vi "TAT_Varient Creater_Station2.vi"(8 "error in (no error)":errorcluster) -> (0 "error out":errorcluster)   [LabVIEW 2017]
uses:
  <vilib>/Utility/miscctls.llb/LVRangeTypeDef.ctl
  <vilib>/addons/database/Connection.llb/Conn ObjectReference.ctl
  <vilib>/Utility/miscctls.llb/LVRowAndColumnUnsignedTypeDef.ctl
  cc04d7d6-45d9-4bf1-9dd6-3a820b5b8d83.vi
  <vilib>/Utility/config.llb/Read Key (I32).vi
  <vilib>/Utility/config.llb/Read Key (String).vi
  <vilib>/Utility/config.llb/Read Key (Boolean).vi
  <vilib>/Utility/config.llb/Write Key (U32).vi
  <vilib>/Utility/config.llb/Write Key (String).vi
  <vilib>/Utility/config.llb/Write Key (Boolean).vi
  <vilib>/Utility/config.llb/NI_LVConfig.lvlib
  <vilib>/addons/database/NI_Database_API.lvlib
panel:
  in  "STATION 1\nBYPASS":bool
  in  "Vertical Slider Control":dbl(slide)=1.0 scale=0.0..-2.0
  in  "CANCLE 3":bool
  in  "PRINTING":bool
  in  "Manual print":bool
  in  "Cancle 2":bool
  in  "Delete Button":bool
  in  "Cancle":bool
  in  "Save Button":bool
  in  "TORISHI CODE":string
  in  "PART NUMBER":string
  in  "Delete Square":bool
  in  "EDIT & SAVE":bool
  out "Varient Details":string[][](table)
  in  "BATCH SIZE":u16=1 min=1 max=100 step=1
  in  "VARIENT NUMBER":u16=1 min=1 max=100 step=1
  in  "HOME":bool
  in  "UPDATE TABLE":bool
  in  "PART NAME":string(combo)
  # "Varient Creater Station 2"
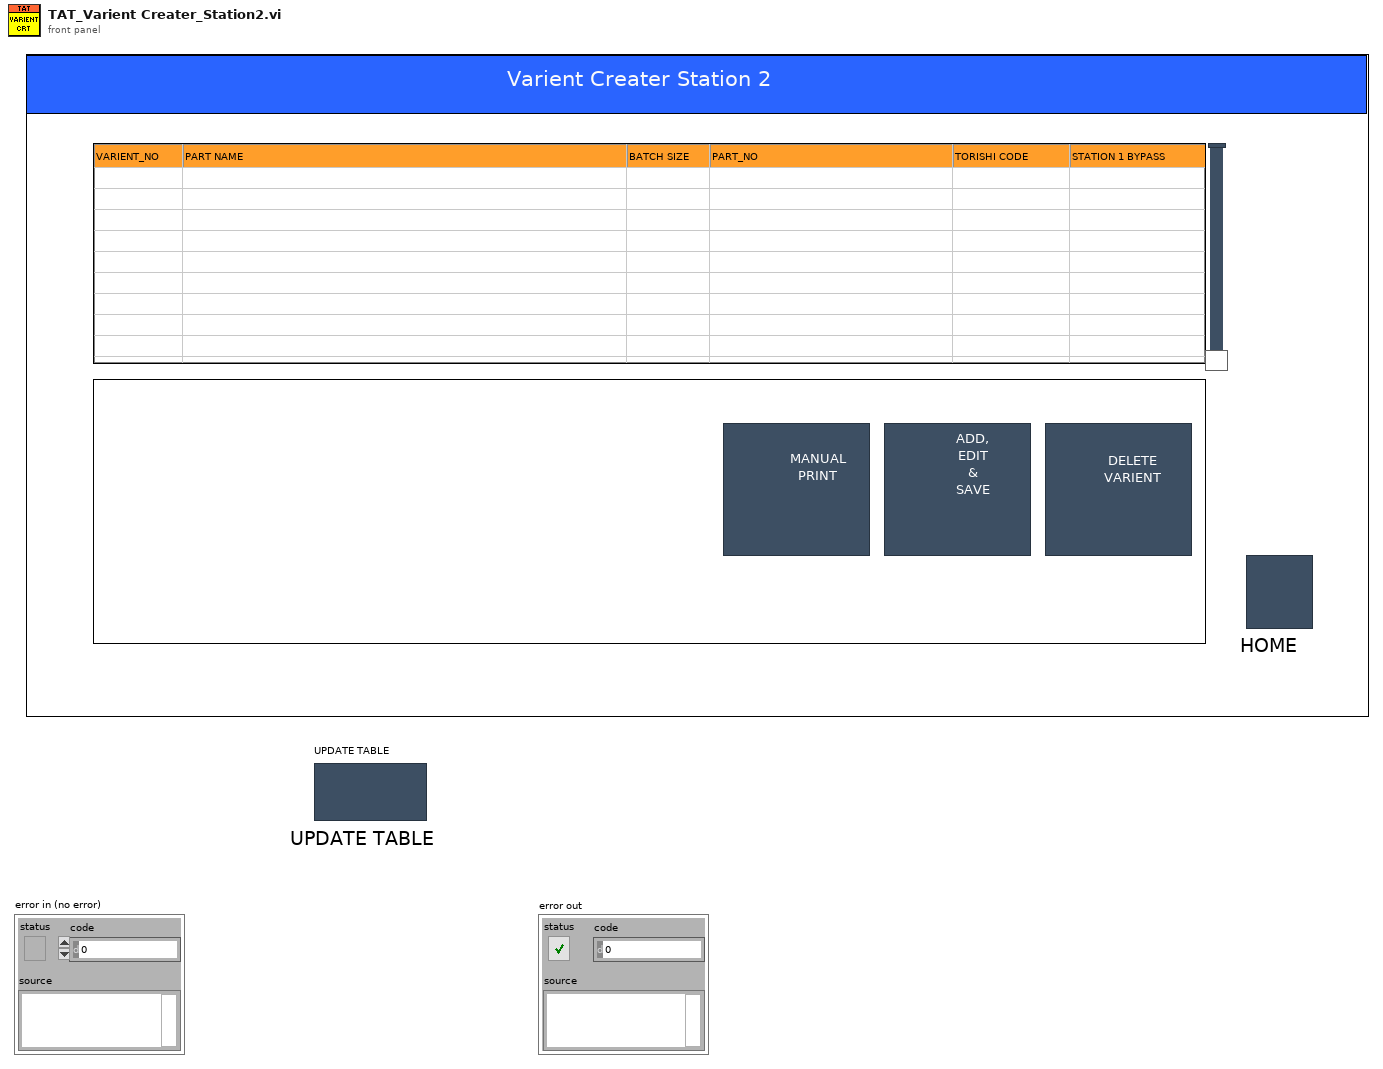
[diagram p1: front panel]
types:
  T1 = enum8{"Enabled", "Disabled", "Disabled and Grayed Out"}
  T2 = enum32{"invalid app kind", "Development System", "Run Time System", "Student Edition", "Embedded LabVIEW", "Evaluation", "Custom"}
  T3 = typedef "NI_LVConfig.lvlib/Config Data RefNum.ctl" = refnum<k1>
  T4 = typedef "LVRangeTypeDef.ctl" = cluster{"Minimum":dbl, "Maximum":dbl, "Increment":dbl, "Minor Increment":dbl, "Start":dbl}
  T5 = typedef "NI_Database_API.lvlib/Conn ObjectReference.ctl" = refnum<k1>
  T6 = cluster{"Varient number":u16, "Part name":string, "connection reference":T5, "Batch_Size":u16, "PART_NO":string, "TORISHI_CODE":string, "scanner com":refnum<visa-resource-name>, "Part Name List":string[], "Varient path":path, "Current Varient path":path, "Communication path":path, "Package path":path, "Part PRN path":path, "Station2 printer IP":string, "Station1 printer IP":string, "Current Serial Number":string, "Station1_QR":string, "Serial_Number":path, "PRIVIOUS code":string[], "Barcode station2 log":string, "Barcode station2 Up":string, "HARNESS CODE":string, "Station 1 Bypass":bool}
  T7 = enum16{"open", "replace", "create", "open or create", "replace or create", "replace or create with confirmation"}
  T8 = typedef "LVRowAndColumnUnsignedTypeDef.ctl" = cluster{"Row":u32, "Column":u32}
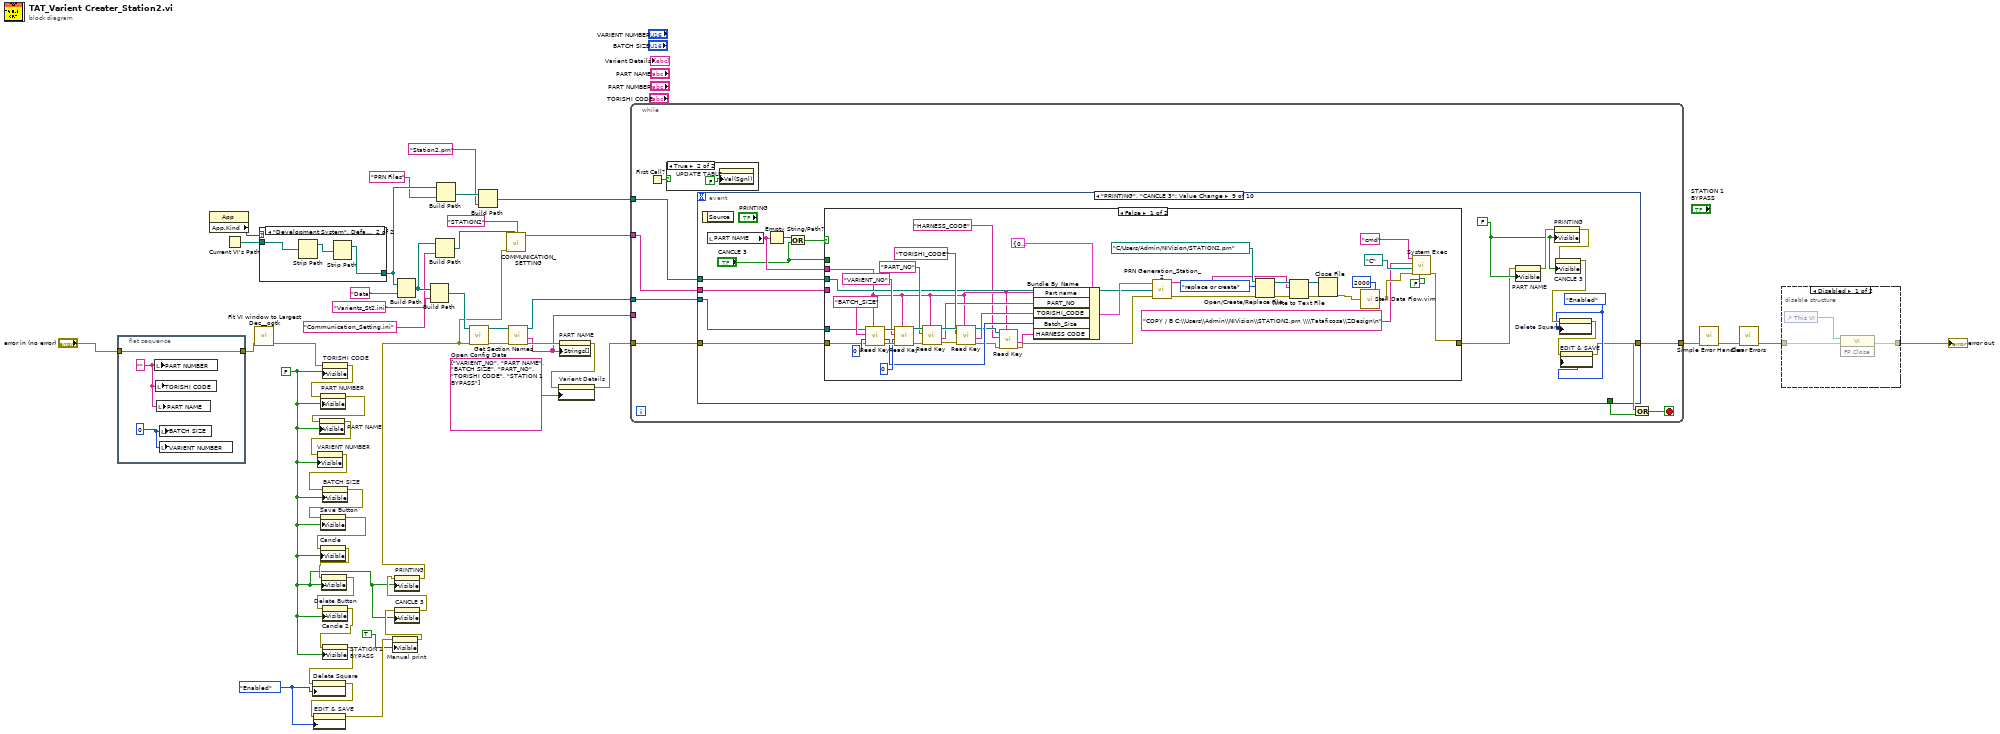
[diagram p0: block diagram]
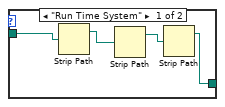
[diagram p3: hidden frame]
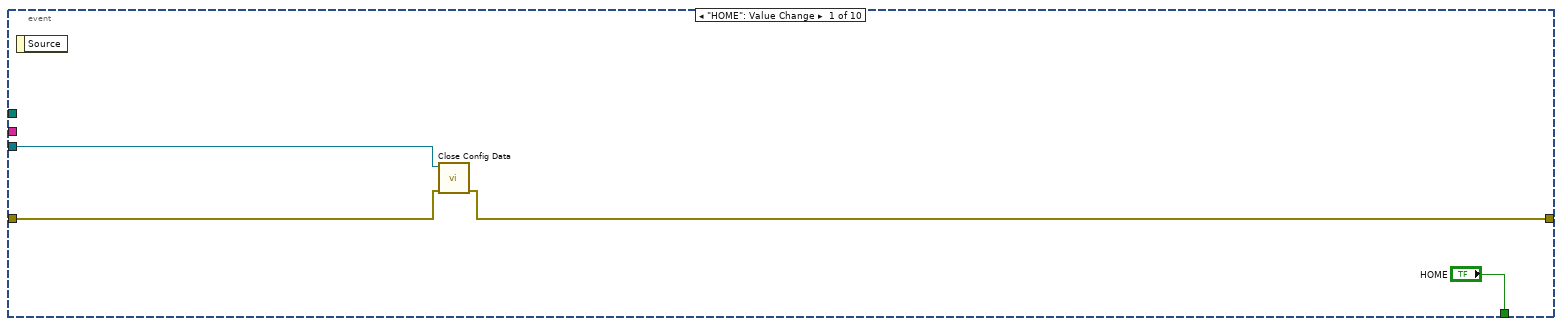
[diagram p5: hidden frame]
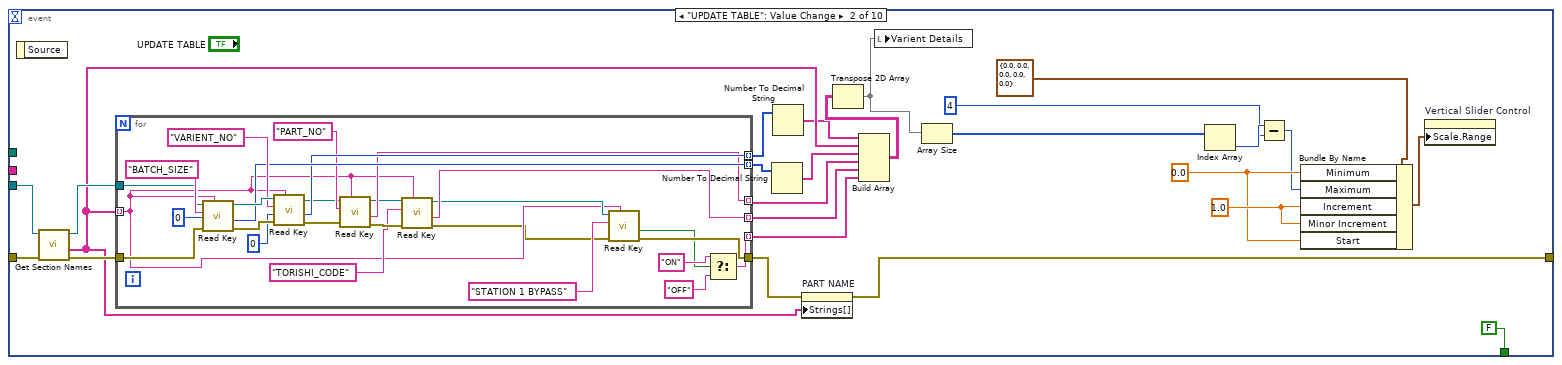
[diagram p6: hidden frame]
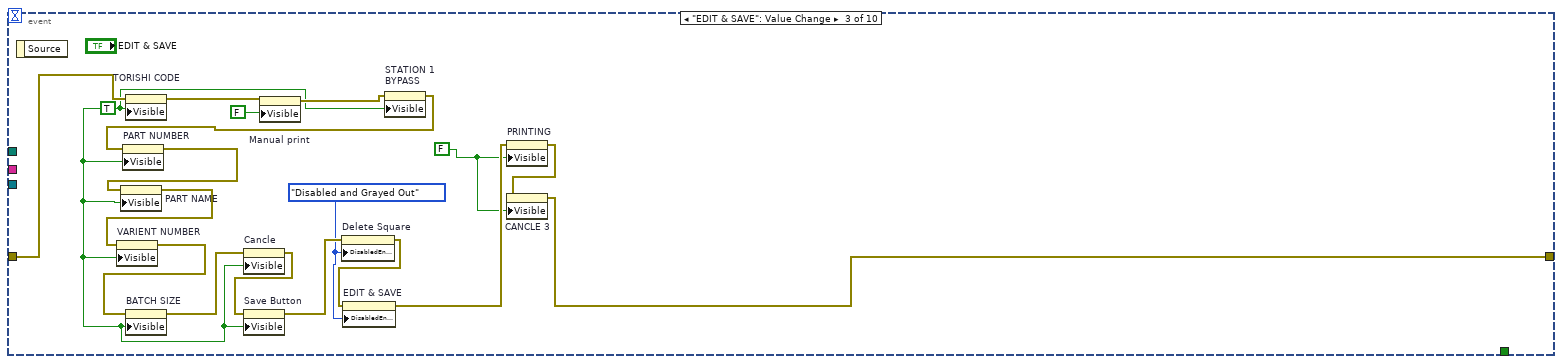
[diagram p7: hidden frame]
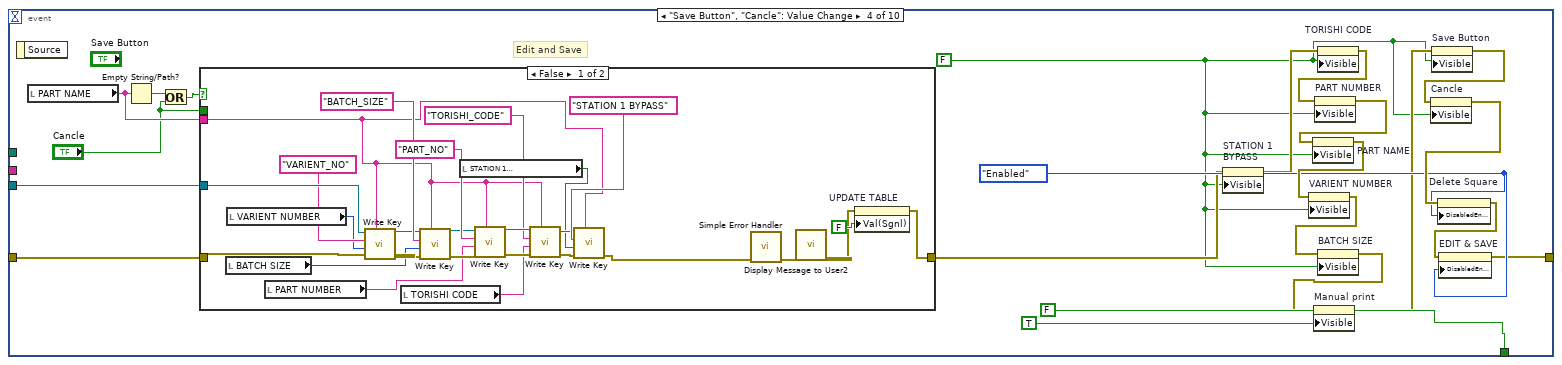
[diagram p8: hidden frame]
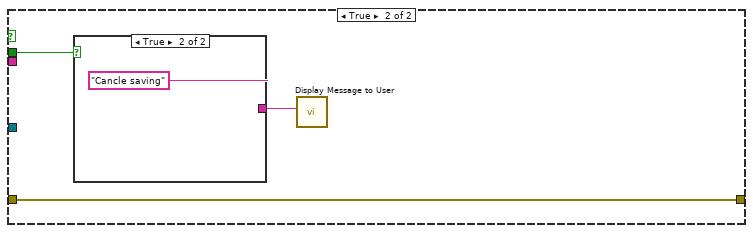
[diagram p9: hidden frame]
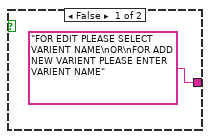
[diagram p10: hidden frame]
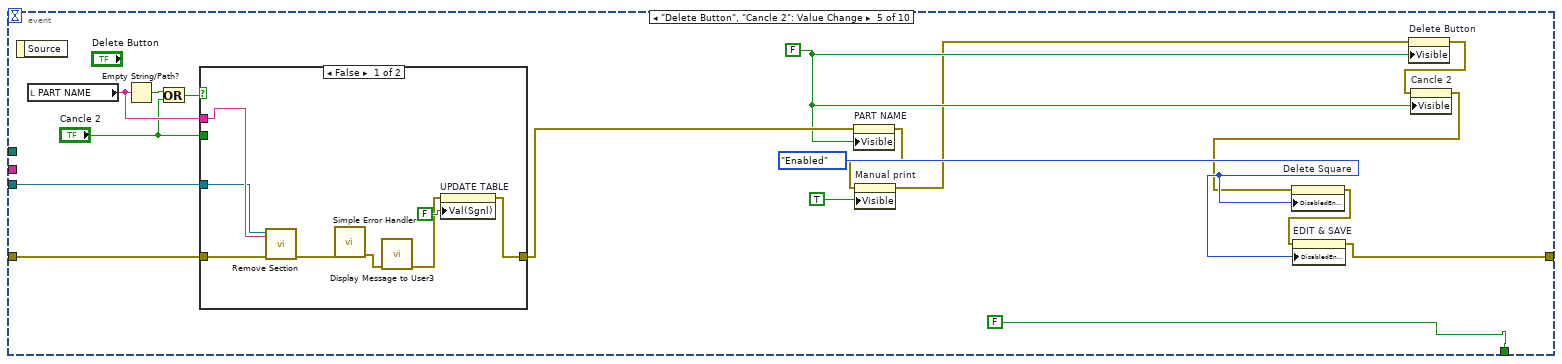
[diagram p11: hidden frame]
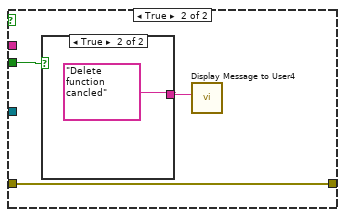
[diagram p12: hidden frame]
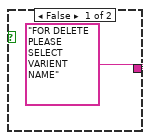
[diagram p13: hidden frame]
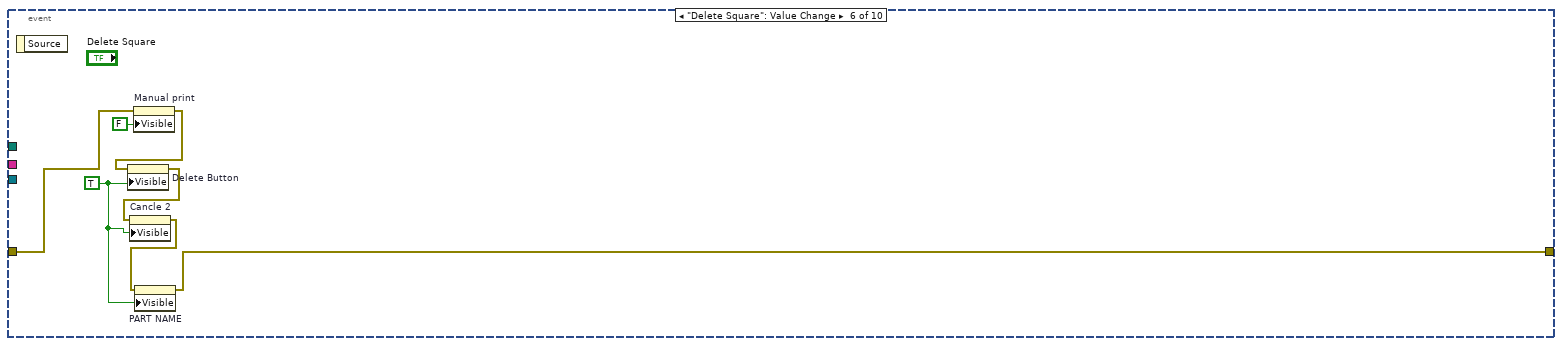
[diagram p14: hidden frame]
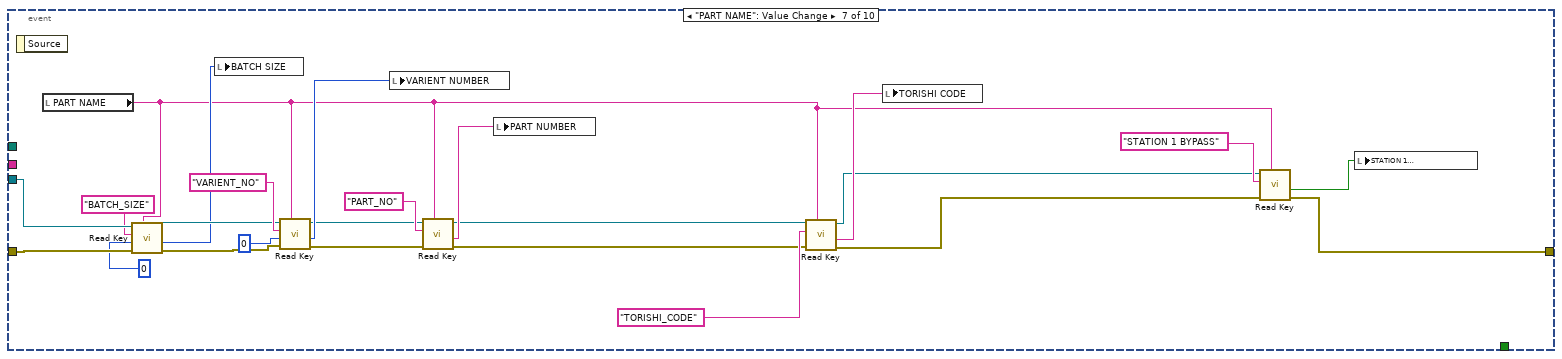
[diagram p15: hidden frame]
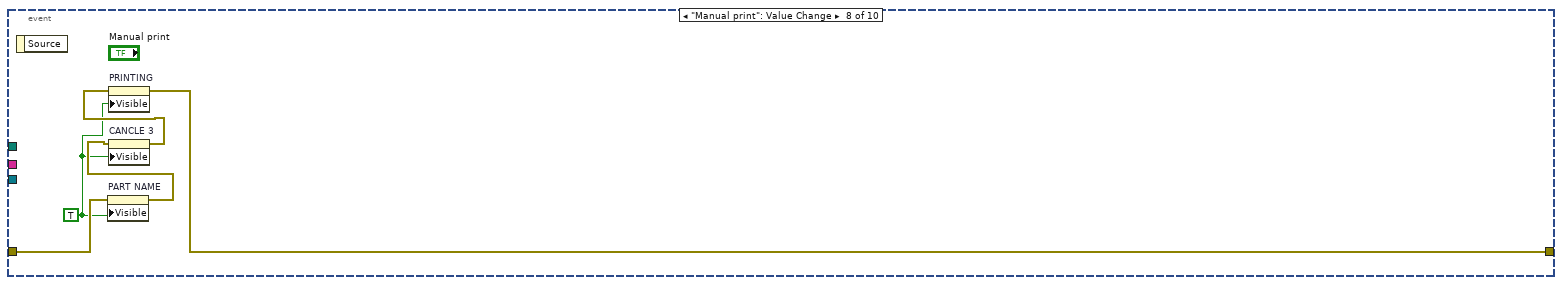
[diagram p16: hidden frame]
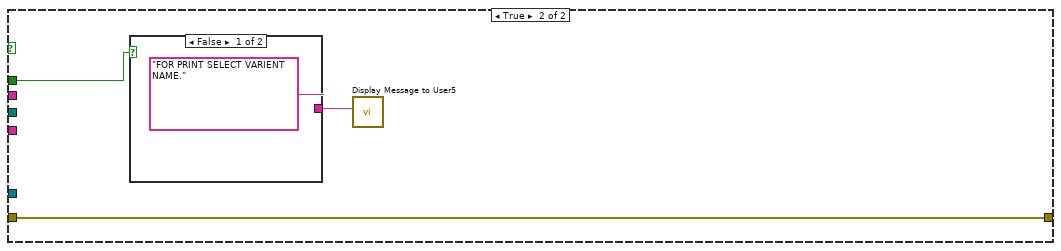
[diagram p17: hidden frame]
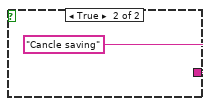
[diagram p18: hidden frame]
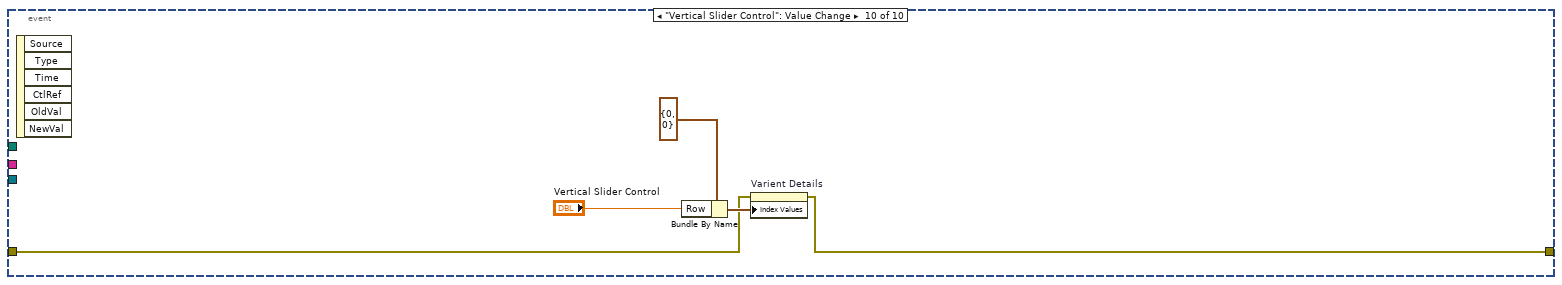
[diagram p19: hidden frame]
diagram:
  w22 = T1."Enabled" ("Disabled")
  w3 = FALSE
  n1 = flat-sequence {
    tunnel: [w49] -> w30
    tunnel: "error in (no error)" -> [w49]
    frame #0 {
      w50 = u16 0 ("BATCH SIZE")
      w51 = "" ("PART NUMBER")
      n2 = local write "PART NUMBER"(w51) -> ()
      n3 = local write "TORISHI CODE"(w51) -> ()
      n4 = local write "PART NAME"(w51) -> ()
      n5 = local write "BATCH SIZE"(w50) -> ()
      n6 = local write "VARIENT NUMBER"(w50) -> ()
    }
  }
  n7 = property class="App"() -> ("App.Kind"=w43:T2)  [unwired: 2 in, 2 out]
  n8 = Current VI's Path() -> (path=w44:path)
  n9 = call <userlib>:"Fit VI window to Largest Dec__ogtk.vi"("error in (no error)"=w30) -> ("error out"=w25:errorcluster)  [unwired: 5 in, 1 out]
  n10 = case shown="\"Development System\", Default" w43 {
    tunnel: w44 -> [w53 w57]
    tunnel: [w52 w56] -> w8
    frame "Run Time System" {
      n11 = Strip Path(path=w53) -> (stripped path=w55:path)  [unwired: 1 out]
      n12 = Strip Path(path=w55) -> (stripped path=w54:path)  [unwired: 1 out]
      n13 = Strip Path(path=w54) -> (stripped path=w52:path)  [unwired: 1 out]
    }
    frame "Development System", Default {
      n14 = Strip Path(path=w57) -> (stripped path=w58:path)  [unwired: 1 out]
      n15 = Strip Path(path=w58) -> (stripped path=w56:path)  [unwired: 1 out]
    }
  }
  n16 = property on="TORISHI CODE" class="Str"(error in=w25, "Visible"=w3) -> (error out=w29:errorcluster)  [unwired: 1 in, 1 out]
  n17 = property on="PART NUMBER" class="Str"(error in=w29, "Visible"=w3) -> (error out=w28:errorcluster)  [unwired: 1 in, 1 out]
  n18 = property on="PART NAME" class="CmbBox"(error in=w28, "Visible"=w3) -> (error out=w27:errorcluster)  [unwired: 1 in, 1 out]
  n19 = property on="VARIENT NUMBER" class="DigNum (strict)"(error in=w27, "Visible"=w3) -> (error out=w26:errorcluster)  [unwired: 1 in, 1 out]
  n20 = property on="BATCH SIZE" class="DigNum (strict)"(error in=w26, "Visible"=w3) -> (error out=w24:errorcluster)  [unwired: 1 in, 1 out]
  n21 = property on="Save Button" class="Bool"(error in=w24, "Visible"=w3) -> (error out=w21:errorcluster)  [unwired: 1 in, 1 out]
  n22 = property on="Cancle" class="Bool"(error in=w21, "Visible"=w3) -> (error out=w20:errorcluster)  [unwired: 1 in, 1 out]
  n23 = property on="Delete Button" class="Bool"(error in=w20, "Visible"=w3) -> (error out=w19:errorcluster)  [unwired: 1 in, 1 out]
  n24 = property on="Cancle 2" class="Bool"(error in=w19, "Visible"=w3) -> (error out=w2:errorcluster)  [unwired: 1 in, 1 out]
  n25 = property on="STATION 1\nBYPASS" class="Bool (strict)"(error in=w2, "Visible"=w3) -> (error out=w1:errorcluster)  [unwired: 1 in, 1 out]
  n26 = property on="Delete Square" class="Bool"(error in=w1, "DisabledEnum"=w22) -> (error out=w23:errorcluster)  [unwired: 1 in, 1 out]
  n27 = property on="EDIT & SAVE" class="Bool"(error in=w23, "DisabledEnum"=w22) -> (error out=w17:errorcluster)  [unwired: 1 in, 1 out]
  n28 = property on="Manual print" class="Bool"(error in=w17, "Visible"=TRUE) -> (error out=w16:errorcluster)  [unwired: 1 in, 1 out]
  n29 = property on="CANCLE 3" class="Bool"(error in=w16, "Visible"=w3) -> (error out=w18:errorcluster)  [unwired: 1 in, 1 out]
  n30 = property on="PRINTING" class="Bool"(error in=w18, "Visible"=w3) -> (error out=w10:errorcluster)  [unwired: 1 in, 1 out]
  n31 = Build Path(base path=w8, name or relative path="Data") -> (appended path=w14:path)
  n32 = Build Path(base path=w14, name or relative path="Varients_St2.ini") -> (appended path=w42:path)
  n33 = Build Path(base path=w14, name or relative path="Communication_Setting.ini") -> (appended path=w11:path)
  n34 = Build Path(base path=w8, name or relative path="PRN Files") -> (appended path=w6:path)
  n35 = call <vilib>:"Open Config Data.vi"("error in (no error)"=w10, "configuration file path"=w42) -> ("error out"=w38:errorcluster, "refnum"=w39:T3)  [unwired: 7 in, 1 out]
  n36 = Build Path(base path=w6, name or relative path="Station2.prn") -> (appended path=w4:path)
  n37 = call "COMMUNICATION_SETTING.vi"("communication path"=w11, "error in"=w10, "STATION"="STATION2") -> ("PRINT_COM"=w9:string)  [unwired: 6 in, 2 out]
  n38 = call <vilib>:"Get Section Names.vi"("error in (no error)"=w38, "refnum"=w39) -> ("error out"=w37:errorcluster, "section names"=w32:string[], "refnum out"=w36:T3)  [unwired: 7 in]
  n39 = property on="PART NAME" class="CmbBox"(error in=w37, "Strings[]"=w32) -> (error out=w35:errorcluster)  [unwired: 1 in, 1 out]
  n40 = property on="Varient Details" class="Tbl (strict)"(error in=w35, "Column Headers[]"=string[] ["VARIENT_NO", "PART NAME", "BATCH SIZE", "PART_NO", "TORISHI CODE", "STATION 1 BYPASS"] ("Column Header Strings[]")) -> (error out=w34:errorcluster)  [unwired: 1 in, 1 out]
  n41 = while {
    tunnel: w34 -> [w65]
    tunnel: [w63] -> w45
    tunnel: w36 -> [w62]
    tunnel: w32 -> [_]
    tunnel: w9 -> [w60]
    tunnel: w4 -> [w59]
    stop <- w64 stop-if-true
    n42 = First Call?() -> (First Call?: T/F=w61:bool)
    n43 = case shown="True" w61 {
      frame False {
      }
      frame True {
        n44 = property on="UPDATE TABLE" class="Bool (strict)"("Val(Sgnl)"=FALSE) -> ()  [unwired: 2 in, 2 out]
      }
    }
    n45 = event shown="[8] \"PRINTING\", \"CANCLE 3\": Value Change" {
      selector: _ -> [_ _ _ _ _ _ _ _ _ _]
      dyn-events: _ -> [_ _ _ _ _ _ _ _ _ _]
      timeout: _ -> [_ _ _ _ _ _ _ _ _ _]
      tunnel: ["HOME" FALSE ("stop") _ FALSE ("stop") FALSE ("stop") _ _ _ _ _] -> w66
      tunnel: w65 -> [w70 w91 w138 w161 w209 w226 w255 w258 w276 w324]
      tunnel: [w69 w83 w128 w148 w201 w229 w238 w257 w265 w325] -> w63
      tunnel: w62 -> [w68 w89 _ w162 w210 _ w254 _ w272 _]
      tunnel: w60 -> [_ _ _ _ _ _ _ _ w263 _]
      tunnel: w59 -> [_ _ _ _ _ _ _ _ w262 _]
      event "HOME": Value Change {
        n46 = event-data() -> ()  [unwired: 1 in, 1 out]
        n47 = call <vilib>:"Close Config Data.vi"("error in (no error)"=w70, "refnum"=w68) -> ("error out"=w69:errorcluster)  [unwired: 8 in, 1 out]
      }
      event "UPDATE TABLE": Value Change {
        w80 = 1.0 ("Increment")
        w79 = 0.0 ("Minimum")
        n48 = event-data() -> ()  [unwired: 1 in, 1 out]
        n49 = call <vilib>:"Get Section Names.vi"("error in (no error)"=w91, "refnum"=w89) -> ("error out"=w90:errorcluster, "section names"=w84:string[], "refnum out"=w88:T3)  [unwired: 7 in]
        n50 = for {
          tunnel: [w105] -> w85
          tunnel: w90 -> [w117]
          tunnel: w84 -> [w98] mode=indexing
          tunnel: w88 -> [w116]
          tunnel: [w115] -> w94 mode=indexing
          tunnel: [w114] -> w95 mode=indexing
          tunnel: [w110] -> w87 mode=indexing
          tunnel: [w106] -> w86 mode=indexing
          tunnel: [w100] -> w73 mode=indexing
          n51 = call-poly <vilib>:"Read Key.vi"("section"=w98, "error in (no error)"=w117, "default value"=0, "key"="BATCH_SIZE", "refnum"=w116) -> ("error out"=w123:errorcluster, "value"=w115:i32, "refnum out"=w122:T3)  [unwired: 3 in, 1 out]
          n52 = call-poly <vilib>:"Read Key.vi"("section"=w98, "error in (no error)"=w123, "default value"=0, "key"="VARIENT_NO", "refnum"=w122) -> ("error out"=w113:errorcluster, "value"=w114:i32, "refnum out"=w111:T3)  [unwired: 3 in, 1 out]
          n53 = call-poly <vilib>:"Read Key.vi"("section"=w98, "error in (no error)"=w113, "key"="PART_NO", "refnum"=w111) -> ("error out"=w109:errorcluster, "value"=w110:string, "refnum out"=w108:T3)  [unwired: 4 in, 1 out]
          n54 = call-poly <vilib>:"Read Key.vi"("section"=w98, "error in (no error)"=w109, "key"="TORISHI_CODE", "refnum"=w108) -> ("error out"=w97:errorcluster, "value"=w106:string, "refnum out"=w99:T3)  [unwired: 4 in, 1 out]
          n55 = call-poly <vilib>:"Read Key.vi"("section"=w98, "error in (no error)"=w97, "key"="STATION 1 BYPASS", "refnum"=w99) -> ("error out"=w105:errorcluster, "value"=w101:bool)  [unwired: 4 in, 2 out]
          n56 = Select(t="ON" ("String"), s=w101, f="OFF" ("String")) -> (s? t:f=w100:string)
        }
        n57 = Number To Decimal String(number=w94) -> (decimal integer string=w93:string[])  [unwired: 1 in]
        n58 = Number To Decimal String(number=w95) -> (decimal integer string=w72:string[])  [unwired: 1 in]
        n59 = property on="PART NAME" class="CmbBox"(error in=w85, "Strings[]"=w84) -> (error out=w83:errorcluster)  [unwired: 1 in, 1 out]
        n60 = Build Array(w72, w84, w93, w87, w86, w73) -> (w92:string[][])
        n61 = Transpose 2D Array(2D array=w92) -> (transposed array=w82:string[][])
        n62 = local write "Varient Details"(w82) -> ()
        n63 = Array Size(array=w82) -> (size(s)=w81:i32[])
        n64 = Index Array(array=w81) -> (element=w76:i32)  [unwired: 1 in]
        n65 = Subtract(x=w76, y=4) -> (x-y=w75:i32)
        n66 = Bundle By Name(cluster=T4 {"Minimum"=0.0, "Maximum"=0.0, "Increment"=0.0, "Minor Increment"=0.0, "Start"=0.0} ("Scale.Range"), "Minimum"=w79, "Maximum"=w75, "Increment"=w80, "Minor Increment"=w80, "Start"=w79) -> (w78:T4)
        n67 = property on="Vertical Slider Control" class="Slide (strict)"("Scale.Range"=w78) -> ()  [unwired: 2 in, 2 out]
      }
      event "EDIT & SAVE": Value Change {
        w127 = FALSE
        w135 = T1."Disabled and Grayed Out" ("Disabled")
        w124 = TRUE
        n68 = event-data() -> ()  [unwired: 1 in, 1 out]
        n69 = property on="TORISHI CODE" class="Str"(error in=w138, "Visible"=w124) -> (error out=w132:errorcluster)  [unwired: 1 in, 1 out]
        n70 = property on="Manual print" class="Bool"(error in=w132, "Visible"=FALSE) -> (error out=w126:errorcluster)  [unwired: 1 in, 1 out]
        n71 = property on="STATION 1\nBYPASS" class="Bool (strict)"(error in=w126, "Visible"=w124) -> (error out=w125:errorcluster)  [unwired: 1 in, 1 out]
        n72 = property on="PART NUMBER" class="Str"(error in=w125, "Visible"=w124) -> (error out=w139:errorcluster)  [unwired: 1 in, 1 out]
        n73 = property on="PART NAME" class="CmbBox"(error in=w139, "Visible"=w124) -> (error out=w140:errorcluster)  [unwired: 1 in, 1 out]
        n74 = property on="VARIENT NUMBER" class="DigNum (strict)"(error in=w140, "Visible"=w124) -> (error out=w141:errorcluster)  [unwired: 1 in, 1 out]
        n75 = property on="BATCH SIZE" class="DigNum (strict)"(error in=w141, "Visible"=w124) -> (error out=w133:errorcluster)  [unwired: 1 in, 1 out]
        n76 = property on="Cancle" class="Bool"(error in=w133, "Visible"=w124) -> (error out=w134:errorcluster)  [unwired: 1 in, 1 out]
        n77 = property on="Save Button" class="Bool"(error in=w134, "Visible"=w124) -> (error out=w137:errorcluster)  [unwired: 1 in, 1 out]
        n78 = property on="Delete Square" class="Bool"(error in=w137, "DisabledEnum"=w135) -> (error out=w136:errorcluster)  [unwired: 1 in, 1 out]
        n79 = property on="EDIT & SAVE" class="Bool"(error in=w136, "DisabledEnum"=w135) -> (error out=w129:errorcluster)  [unwired: 1 in, 1 out]
        n80 = property on="PRINTING" class="Bool"(error in=w129, "Visible"=w127) -> (error out=w130:errorcluster)  [unwired: 1 in, 1 out]
        n81 = property on="CANCLE 3" class="Bool"(error in=w130, "Visible"=w127) -> (error out=w128:errorcluster)  [unwired: 1 in, 1 out]
      }
      event "Save Button", "Cancle": Value Change {
        w149 = T1."Enabled" ("Disabled")
        w142 = FALSE
        # "Edit and Save"
        n82 = event-data() -> ()  [unwired: 1 in, 1 out]
        n83 = local read "PART NAME"() -> (w160:string)
        n84 = Empty String/Path?(string/path=w160) -> (empty?=w159:bool)
        n85 = Or(x=w159, y="Cancle") -> (x .or. y?=w158:bool)
        n86 = case shown="False" w158 {
          tunnel: w161 -> [w188 w192]
          tunnel: [w182 w192] -> w144
          tunnel: w162 -> [w186 _]
          tunnel: w160 -> [w165 _]
          tunnel: "Cancle" -> [_ w190]
          frame False {
            n87 = local read "BATCH SIZE"() -> (w181:u16)
            n88 = local read "VARIENT NUMBER"() -> (w180:u16)
            n89 = local read "PART NUMBER"() -> (w170:string)
            n90 = call-poly <vilib>:"Write Key.vi"("section"=w165, "error in (no error)"=w188, "value"=w180, "key"="VARIENT_NO", "refnum"=w186) -> ("error out"=w187:errorcluster, "refnum out"=w185:T3)  [unwired: 4 in, 1 out]
            n91 = local read "TORISHI CODE"() -> (w171:string)
            n92 = call-poly <vilib>:"Write Key.vi"("section"=w165, "error in (no error)"=w187, "value"=w181, "key"="BATCH_SIZE", "refnum"=w185) -> ("error out"=w175:errorcluster, "refnum out"=w173:T3)  [unwired: 4 in, 1 out]
            n93 = local read "STATION 1\nBYPASS"() -> (w166:bool)
            n94 = call-poly <vilib>:"Write Key.vi"("section"=w165, "error in (no error)"=w175, "value"=w170, "key"="PART_NO", "refnum"=w173) -> ("error out"=w176:errorcluster, "refnum out"=w177:T3)  [unwired: 4 in, 1 out]
            n95 = call-poly <vilib>:"Write Key.vi"("section"=w165, "error in (no error)"=w176, "value"=w171, "key"="TORISHI_CODE", "refnum"=w177) -> ("error out"=w168:errorcluster, "refnum out"=w167:T3)  [unwired: 4 in, 1 out]
            n96 = call-poly <vilib>:"Write Key.vi"("section"=w165, "error in (no error)"=w168, "value"=w166, "key"="STATION 1 BYPASS", "refnum"=w167) -> ("error out"=w164:errorcluster)  [unwired: 4 in, 2 out]
            n97 = call <vilib>:"Simple Error Handler.vi"("error in (no error)"=w164) -> ("error out"=w179:errorcluster)  [unwired: 4 in, 4 out]
            n98 = call "Display Message to User2"("error in (no error)"=w179) -> ("error out"=w178:errorcluster)  [unwired: 9 in, 1 out]
            n99 = property on="UPDATE TABLE" class="Bool (strict)"(error in=w178, "Val(Sgnl)"=FALSE) -> (error out=w182:errorcluster)  [unwired: 1 in, 1 out]
          }
          frame True {
            n100 = case shown="True" w190 {
              tunnel: ["FOR EDIT PLEASE SELECT VARIENT NAME\nOR\nFOR ADD NEW VARIENT PLEASE ENTER VARIENT NAME" "Cancle saving"] -> w191
              frame False {
              }
              frame True {
              }
            }
            n101 = call "Display Message to User"("Message"=w191) -> ()  [unwired: 9 in, 2 out]
          }
        }
        n102 = property on="STATION 1\nBYPASS" class="Bool (strict)"(error in=w144, "Visible"=w142) -> (error out=w143:errorcluster)  [unwired: 1 in, 1 out]
        n103 = property on="TORISHI CODE" class="Str"(error in=w143, "Visible"=w142) -> (error out=w156:errorcluster)  [unwired: 1 in, 1 out]
        n104 = property on="PART NUMBER" class="Str"(error in=w156, "Visible"=w142) -> (error out=w155:errorcluster)  [unwired: 1 in, 1 out]
        n105 = property on="PART NAME" class="CmbBox"(error in=w155, "Visible"=w142) -> (error out=w154:errorcluster)  [unwired: 1 in, 1 out]
        n106 = property on="VARIENT NUMBER" class="DigNum (strict)"(error in=w154, "Visible"=w142) -> (error out=w153:errorcluster)  [unwired: 1 in, 1 out]
        n107 = property on="BATCH SIZE" class="DigNum (strict)"(error in=w153, "Visible"=w142) -> (error out=w146:errorcluster)  [unwired: 1 in, 1 out]
        n108 = property on="Manual print" class="Bool"(error in=w146, "Visible"=TRUE) -> (error out=w145:errorcluster)  [unwired: 1 in, 1 out]
        n109 = property on="Save Button" class="Bool"(error in=w145, "Visible"=w142) -> (error out=w151:errorcluster)  [unwired: 1 in, 1 out]
        n110 = property on="Cancle" class="Bool"(error in=w151, "Visible"=w142) -> (error out=w150:errorcluster)  [unwired: 1 in, 1 out]
        n111 = property on="Delete Square" class="Bool"(error in=w150, "DisabledEnum"=w149) -> (error out=w152:errorcluster)  [unwired: 1 in, 1 out]
        n112 = property on="EDIT & SAVE" class="Bool"(error in=w152, "DisabledEnum"=w149) -> (error out=w148:errorcluster)  [unwired: 1 in, 1 out]
      }
      event "Delete Button", "Cancle 2": Value Change {
        w203 = T1."Enabled" ("Disabled")
        w198 = FALSE
        n113 = event-data() -> ()  [unwired: 1 in, 1 out]
        n114 = local read "PART NAME"() -> (w208:string)
        n115 = Empty String/Path?(string/path=w208) -> (empty?=w207:bool)
        n116 = Or(x=w207, y="Cancle 2") -> (x .or. y?=w206:bool)
        n117 = case shown="False" w206 {
          tunnel: w209 -> [w213 w222]
          tunnel: [w218 w222] -> w202
          tunnel: w210 -> [w214 _]
          tunnel: w208 -> [w215 _]
          tunnel: "Cancle 2" -> [_ w221]
          frame False {
            n118 = call <vilib>:"Remove Section.vi"("section"=w215, "error in (no error)"=w213, "refnum"=w214) -> ("error out"=w212:errorcluster)  [unwired: 6 in, 2 out]
            n119 = call <vilib>:"Simple Error Handler.vi"("error in (no error)"=w212) -> ("error out"=w217:errorcluster)  [unwired: 4 in, 4 out]
            n120 = call "Display Message to User3"("error in (no error)"=w217) -> ("error out"=w216:errorcluster)  [unwired: 9 in, 1 out]
            n121 = property on="UPDATE TABLE" class="Bool (strict)"(error in=w216, "Val(Sgnl)"=FALSE) -> (error out=w218:errorcluster)  [unwired: 1 in, 1 out]
          }
          frame True {
            n122 = case shown="True" w221 {
              tunnel: ["FOR DELETE PLEASE SELECT VARIENT NAME" "Delete function cancled"] -> w220
              frame False {
              }
              frame True {
              }
            }
            n123 = call "Display Message to User4"("Message"=w220) -> ()  [unwired: 9 in, 2 out]
          }
        }
        n124 = property on="PART NAME" class="CmbBox"(error in=w202, "Visible"=w198) -> (error out=w196:errorcluster)  [unwired: 1 in, 1 out]
        n125 = property on="Manual print" class="Bool"(error in=w196, "Visible"=TRUE) -> (error out=w195:errorcluster)  [unwired: 1 in, 1 out]
        n126 = property on="Delete Button" class="Bool"(error in=w195, "Visible"=w198) -> (error out=w200:errorcluster)  [unwired: 1 in, 1 out]
        n127 = property on="Cancle 2" class="Bool"(error in=w200, "Visible"=w198) -> (error out=w199:errorcluster)  [unwired: 1 in, 1 out]
        n128 = property on="Delete Square" class="Bool"(error in=w199, "DisabledEnum"=w203) -> (error out=w204:errorcluster)  [unwired: 1 in, 1 out]
        n129 = property on="EDIT & SAVE" class="Bool"(error in=w204, "DisabledEnum"=w203) -> (error out=w201:errorcluster)  [unwired: 1 in, 1 out]
      }
      event "Delete Square": Value Change {
        w228 = TRUE
        n130 = event-data() -> ()  [unwired: 1 in, 1 out]
        n131 = property on="Manual print" class="Bool"(error in=w226, "Visible"=FALSE) -> (error out=w225:errorcluster)  [unwired: 1 in, 1 out]
        n132 = property on="Delete Button" class="Bool"(error in=w225, "Visible"=w228) -> (error out=w231:errorcluster)  [unwired: 1 in, 1 out]
        n133 = property on="Cancle 2" class="Bool"(error in=w231, "Visible"=w228) -> (error out=w230:errorcluster)  [unwired: 1 in, 1 out]
        n134 = property on="PART NAME" class="CmbBox"(error in=w230, "Visible"=w228) -> (error out=w229:errorcluster)  [unwired: 1 in, 1 out]
      }
      event "PART NAME": Value Change {
        n135 = event-data() -> ()  [unwired: 1 in, 1 out]
        n136 = local read "PART NAME"() -> (w232:string)
        n137 = call-poly <vilib>:"Read Key.vi"("section"=w232, "error in (no error)"=w255, "default value"=0, "key"="BATCH_SIZE", "refnum"=w254) -> ("error out"=w251:errorcluster, "value"=w246:i32, "refnum out"=w250:T3)  [unwired: 3 in, 1 out]
        n138 = local write "BATCH SIZE"(w246) -> ()
        n139 = call-poly <vilib>:"Read Key.vi"("section"=w232, "error in (no error)"=w251, "default value"=0, "key"="VARIENT_NO", "refnum"=w250) -> ("error out"=w245:errorcluster, "value"=w249:i32, "refnum out"=w242:T3)  [unwired: 3 in, 1 out]
        n140 = local write "VARIENT NUMBER"(w249) -> ()
        n141 = call-poly <vilib>:"Read Key.vi"("section"=w232, "error in (no error)"=w245, "key"="PART_NO", "refnum"=w242) -> ("error out"=w234:errorcluster, "value"=w241:string, "refnum out"=w233:T3)  [unwired: 4 in, 1 out]
        n142 = local write "PART NUMBER"(w241) -> ()
        n143 = call-poly <vilib>:"Read Key.vi"("section"=w232, "error in (no error)"=w234, "key"="TORISHI_CODE", "refnum"=w233) -> ("error out"=w239:errorcluster, "value"=w240:string, "refnum out"=w236:T3)  [unwired: 4 in, 1 out]
        n144 = local write "TORISHI CODE"(w240) -> ()
        n145 = call-poly <vilib>:"Read Key.vi"("section"=w232, "error in (no error)"=w239, "key"="STATION 1 BYPASS", "refnum"=w236) -> ("error out"=w238:errorcluster, "value"=w235:bool)  [unwired: 4 in, 2 out]
        n146 = local write "STATION 1\nBYPASS"(w235) -> ()
      }
      event "Manual print": Value Change {
        w256 = TRUE
        n147 = event-data() -> ()  [unwired: 1 in, 1 out]
        n148 = property on="PART NAME" class="CmbBox"(error in=w258, "Visible"=w256) -> (error out=w260:errorcluster)  [unwired: 1 in, 1 out]
        n149 = property on="CANCLE 3" class="Bool"(error in=w260, "Visible"=w256) -> (error out=w259:errorcluster)  [unwired: 1 in, 1 out]
        n150 = property on="PRINTING" class="Bool"(error in=w259, "Visible"=w256) -> (error out=w257:errorcluster)  [unwired: 1 in, 1 out]
      }
      event "PRINTING", "CANCLE 3": Value Change {
        w266 = T1."Enabled" ("Disabled")
        w267 = FALSE
        n151 = event-data() -> ()  [unwired: 1 in, 1 out]
        n152 = local read "PART NAME"() -> (w273:string)
        n153 = Empty String/Path?(string/path=w273) -> (empty?=w275:bool)
        n154 = Or(x=w275, y="CANCLE 3") -> (x .or. y?=w274:bool)
        n155 = case shown="False" w274 {
          tunnel: w276 -> [w307 w321]
          tunnel: [w280 w321] -> w264
          tunnel: w273 -> [w296 _]
          tunnel: w272 -> [w306 _]
          tunnel: w263 -> [_ _]
          tunnel: w262 -> [w300 _]
          tunnel: "CANCLE 3" -> [_ w319]
          frame False {
            n156 = call-poly <vilib>:"Read Key.vi"("section"=w296, "error in (no error)"=w307, "default value"=0, "key"="BATCH_SIZE", "refnum"=w306) -> ("error out"=w318:errorcluster, "value"=w304:i32, "refnum out"=w317:T3)  [unwired: 3 in, 1 out]
            n157 = call-poly <vilib>:"Read Key.vi"("section"=w296, "error in (no error)"=w318, "default value"=0, "key"="VARIENT_NO", "refnum"=w317) -> ("error out"=w314:errorcluster, "refnum out"=w313:T3)  [unwired: 3 in, 2 out]
            n158 = call-poly <vilib>:"Read Key.vi"("section"=w296, "error in (no error)"=w314, "key"="PART_NO", "refnum"=w313) -> ("error out"=w315:errorcluster, "value"=w302:string, "refnum out"=w316:T3)  [unwired: 4 in, 1 out]
            n159 = call-poly <vilib>:"Read Key.vi"("section"=w296, "error in (no error)"=w315, "key"="TORISHI_CODE", "refnum"=w316) -> ("error out"=w298:errorcluster, "value"=w305:string, "refnum out"=w297:T3)  [unwired: 4 in, 1 out]
            n160 = call-poly <vilib>:"Read Key.vi"("section"=w296, "error in (no error)"=w298, "key"="HARNESS_CODE", "refnum"=w297) -> ("error out"=w299:errorcluster, "value"=w295:string)  [unwired: 4 in, 2 out]
            n161 = Bundle By Name(cluster=T6 {"Varient number"=0, "Part name"="", "connection reference"=refnum, "Batch_Size"=0, "PART_NO"="", "TORISHI_CODE"="", "scanner com"="", "Part Name List"=[], "Varient path"=path "", "Current Varient path"=path "", "Communication path"=path "", "Package path"=path "", "Part PRN path"=path "", "Station2 printer IP"="", "Station1 printer IP"="", "Current Serial Number"="", "Station1_QR"="", "Serial_Number"=path "", "PRIVIOUS code"=[], "Barcode station2 log"="", "Barcode station2 Up"="", "HARNESS CODE"="", "Station 1 Bypass"=FALSE} ("Cluster 2"), "Part name"=w296, "PART_NO"=w302, "TORISHI_CODE"=w305, "Batch_Size"=w304, "HARNESS CODE"=w295) -> (w301:T6)
            n162 = call "PRN Generation_Station_2.vi"("error in (no error)"=w299, "PRN path"=w300, "Cluster"=w301) -> ("error out"=w279:errorcluster, "PRN to Print"=w278:string)  [unwired: 2 in, 2 out]
            n163 = Open/Create/Replace File(file path (use dialog)=path "C:/Users/Admin/NIVision/STATION2.prn", error in=w279, operation (0:open)=T7."replace or create") -> (refnum out=w291:refnum<file>, error out=w290:errorcluster)  [unwired: 3 in, 1 out]
            n164 = Write to Text File(file (use dialog)=w291, text=w278, error in=w290) -> (refnum out=w289:refnum<file>, error out=w288:errorcluster)  [unwired: 1 in, 1 out]
            n165 = Close File(refnum=w289, error in=w288) -> (error out=w292:errorcluster)  [unwired: 1 out]
            n166 = call "Stall Data Flow.vim"("value in"=w292, "milliseconds to wait"=u32 2000) -> ("value out"=w293:errorcluster)  [unwired: 1 out]
            n167 = call <vilib>:"System Exec.vi"("run minimized? (F)"=FALSE, "error in (no error)"=w293, "working directory"=path "C:/", "standard input"="COPY / B C:\\Users\\Admin\\NIVision\\STATION2.prn \\\\Tataficosa\\ZDesign\n", "command line"="cmd") -> ("error out"=w280:errorcluster)  [unwired: 3 in, 3 out]
          }
          frame True {
            n168 = case shown="False" w319 {
              tunnel: ["FOR PRINT SELECT VARIENT NAME." "Cancle saving"] -> w320
              frame False {
              }
              frame True {
              }
            }
            n169 = call "Display Message to User5"("Message"=w320) -> ()  [unwired: 9 in, 2 out]
          }
        }
        n170 = property on="PART NAME" class="CmbBox"(error in=w264, "Visible"=w267) -> (error out=w271:errorcluster)  [unwired: 1 in, 1 out]
        n171 = property on="PRINTING" class="Bool"(error in=w271, "Visible"=w267) -> (error out=w269:errorcluster)  [unwired: 1 in, 1 out]
        n172 = property on="CANCLE 3" class="Bool"(error in=w269, "Visible"=w267) -> (error out=w268:errorcluster)  [unwired: 1 in, 1 out]
        n173 = property on="Delete Square" class="Bool"(error in=w268, "DisabledEnum"=w266) -> (error out=w270:errorcluster)  [unwired: 1 in, 1 out]
        n174 = property on="EDIT & SAVE" class="Bool"(error in=w270, "DisabledEnum"=w266) -> (error out=w265:errorcluster)  [unwired: 1 in, 1 out]
      }
      event "Vertical Slider Control": Value Change {
        n175 = event-data() -> ()  [unwired: 1 in, 6 out]
        n176 = Bundle By Name(cluster=T8 {"Row"=0, "Column"=0} ("Index Values"), "Row"="Vertical Slider Control") -> (w327:T8)
        n177 = property on="Varient Details" class="Tbl (strict)"(error in=w324, "Index Values"=w327) -> (error out=w325:errorcluster)  [unwired: 1 in, 1 out]
      }
    }
    n178 = Or(x=w63, y=w66) -> (x .or. y?=w64:bool)
  }
  n179 = call <vilib>:"Simple Error Handler.vi"("error in (no error)"=w45) -> ("error out"=w48:errorcluster)  [unwired: 4 in, 4 out]
  n180 = call <vilib>:"Clear Errors.vi"("error in (no error)"=w48) -> ("error out"=w47:errorcluster)  [unwired: 5 in, 1 out]
  n181 = disable-structure shown="Disabled" {
    disable-tunnel: w47 -> [w331 w332]
    disable-tunnel: [w330 w332] -> w46
    frame Disabled {
      n182 = control-ref of="This VI"() -> (w329:refnum<vi>)
      n183 = invoke class="VI" method="FP.Close"(reference=w329, error in=w331) -> (error out=w330:errorcluster)  [unwired: 1 in, 2 out]
    }
    frame Enabled {
    }
  }
  "error out" <- w46
